vi "CANFrame Duration.vi"(8 "error in (no error)":errorcluster, 10 "CAN frame":T1 {"payload" format="%x"; "timestamp" format="%<%.7X\n%x>T"; "type" items=["CAN Data"=0, "CAN Remote"=1, "CAN Bus Error"=2, "CAN 2.0 Data"=8, "CAN FD Data"=16, "CAN FD+BRS Data"=24, "J1939 Data"=192, "Delay"=224, "Log Trigger"=225, "Start Trigger"=226]; "identifier" format="%x"}, 11 "CANBus_Load_Calculator in":refnum<class "CANBus_Load_Calculator.lvclass">) -> (0 "error out":errorcluster, 2 "Frame Duration (us)":u64, 3 "CANBus_Load_Calculator out":refnum<class "CANBus_Load_Calculator.lvclass">)   [LabVIEW 2019, in "XNET-Bus-Load-Calculator.lvlib" / "CANBus_Load_Calculator.lvclass"]
uses:
  CANBus_Load_Calculator.lvclass
  <vilib>/xnet/xnet.llb/XNET Frame CAN.ctl
  <vilib>/xnet/xnet.llb/XNET Frame Type CAN.ctl
  CANBus_Load_Calculator.lvclass/CANBus_Load_Calculator.ctl
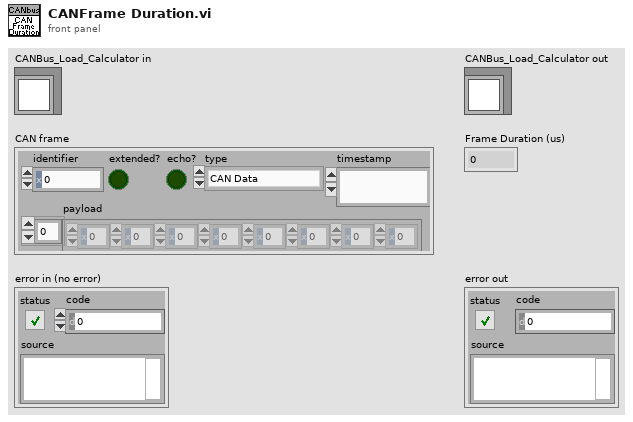
[diagram p1: front panel]
types:
  T1 = typedef "XNET Frame CAN.ctl" = cluster{"timestamp":timestamp, "payload":u8[], "identifier":u32, "type":T2, "extended?":bool, "echo?":bool}
  T2 = typedef "XNET Frame Type CAN.ctl" = u8
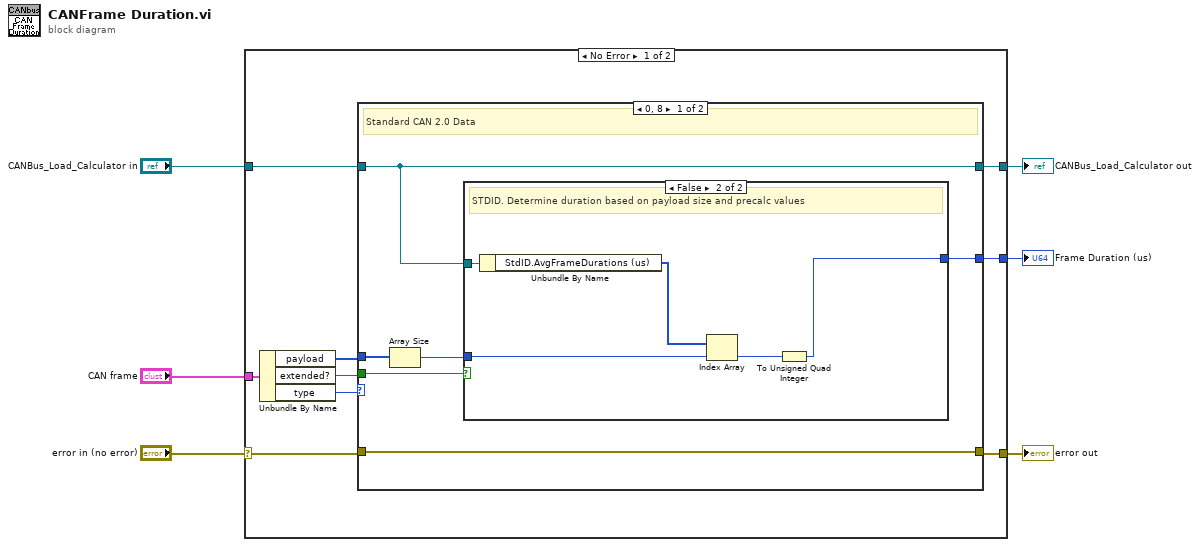
[diagram p0: block diagram]
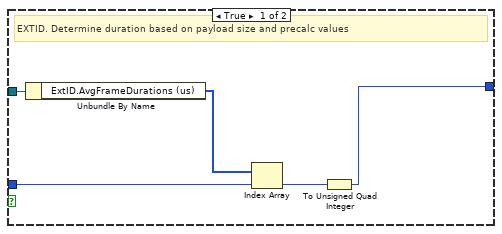
[diagram p2: hidden frame]
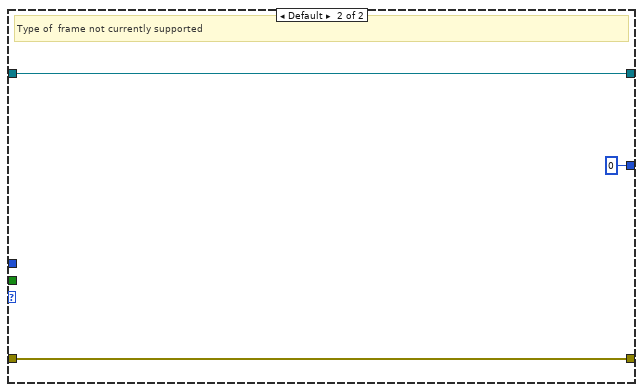
[diagram p3: hidden frame]
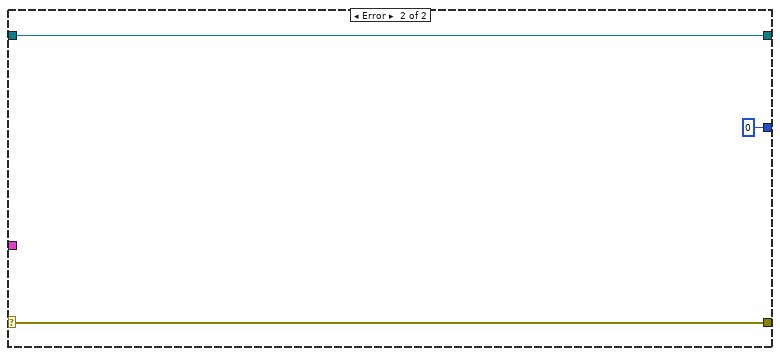
[diagram p4: hidden frame]
diagram:
  n1 = case shown="No Error" "error in (no error)" {
    selector: "error in (no error)" -> [w7 w37]
    tunnel: [w15 u64 0] -> w6
    tunnel: "CANBus_Load_Calculator in" -> [w12 w35]
    tunnel: [w11 w35] -> w4
    tunnel: [w9 w37] -> w3
    tunnel: "CAN frame" -> [w8 _]
    frame No Error {
      n2 = Unbundle By Name(w8) -> ("payload"=w14:u8[], "extended?"=w10:bool, "type"=w13:T2)
      n3 = case shown="0, 8" w13 {
        tunnel: [w21 w34] -> w9
        tunnel: w7 -> [w21 w34]
        tunnel: w10 -> [w20 _]
        tunnel: [w17 w33] -> w11
        tunnel: w12 -> [w17 w33]
        tunnel: w14 -> [w19 _]
        tunnel: [w16 u64 0] -> w15
        frame 0, 8 {
          # "Standard CAN 2.0 Data"
          n4 = Array Size(array=w19) -> (size(s)=w18:i32)
          n5 = case shown="False" w20 {
            tunnel: w18 -> [w24 w29]
            tunnel: w17 -> [w26 w31]
            tunnel: [w22 w27] -> w16
            frame True {
              # "EXTID. Determine duration based on payload size and precalc values"
              n6 = Unbundle By Name(w26) -> ("ExtID.AvgFrameDurations (us)"=w25:u32[])
              n7 = Index Array "Index Array"(array=w25, index=w24) -> (element=w23:u32)
              n8 = To Unsigned Quad Integer(1:w23) -> (0:w22:u64)
            }
            frame False {
              # "STDID. Determine duration based on payload size and precalc values"
              n9 = Unbundle By Name(w31) -> ("StdID.AvgFrameDurations (us)"=w30:u32[])
              n10 = Index Array "Index Array"(array=w30, index=w29) -> (element=w28:u32)
              n11 = To Unsigned Quad Integer(1:w28) -> (0:w27:u64)
            }
          }
        }
        frame Default {
          # "Type of  frame not currently supported"
        }
      }
    }
    frame Error {
    }
  }
  "Frame Duration (us)" <- w6
  "CANBus_Load_Calculator out" <- w4
  "error out" <- w3
